vi "transferPrivate.vi"(8 "error in (no error)":errorcluster, 10 "TransferFrom in":refnum<class "xceNode.lvclass">, 11 "TransferTo in":refnum<class "xceDataNode.lvclass">) -> (0 "error out":errorcluster, 2 "TransferFrom out":refnum<class "xceNode.lvclass">, 3 "TransferTo out":refnum<class "xceDataNode.lvclass">)   [LabVIEW 2013, in "xceDataNode.lvclass"]
doc: "Transfers all private data from one xceDataNode to another. Used primarily to replace a node with another in the tree data structure."
uses:
  xceDataNode.lvclass
  xceNode/xceNode.lvclass
  xceDataNode.lvclass/xceDataNode.ctl
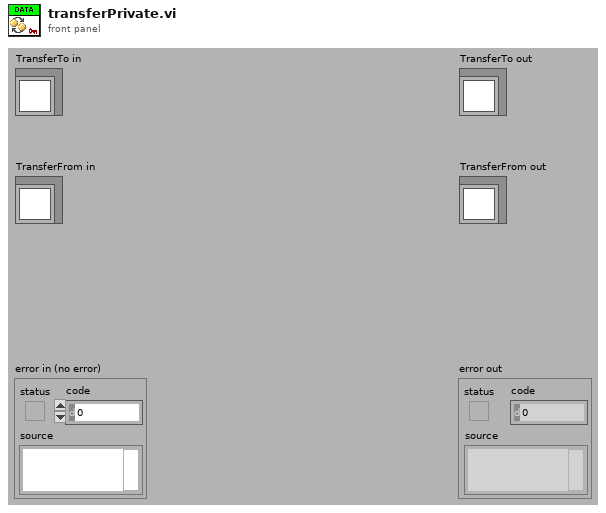
[diagram p1: front panel]
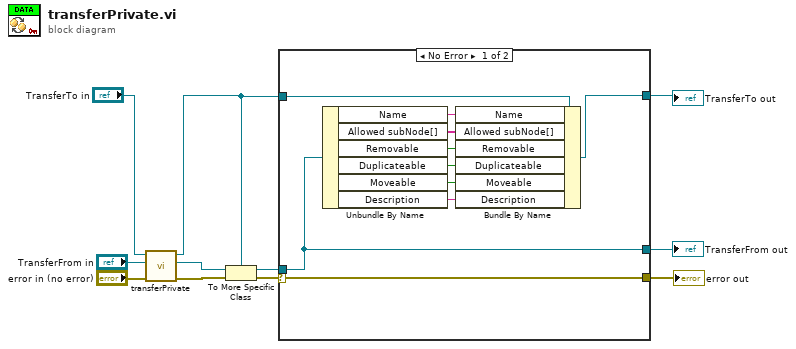
[diagram p0: block diagram]
diagram:
  n1 = call-parent "transferPrivate.vi"("error in (no error)"="error in (no error)", "TransferFrom in"="TransferFrom in", "TransferTo in"="TransferTo in") -> ("error out"=w7:errorcluster, "TransferFrom out"=w8:refnum<class "xceNode.lvclass">, "TransferTo out"=w5:refnum<class "xceDataNode.lvclass">)  [unwired: 6 in]
  n2 = To More Specific Class(target class=w5, reference=w8, error in=w7) -> (specific class reference=w4:refnum<class "xceDataNode.lvclass">, error out=w6:errorcluster)
  n3 = case shown="No Error" w6 {
    selector: w6 -> [w14 w22]
    tunnel: w5 -> [w21 w24]
    tunnel: w4 -> [w13 w23]
    tunnel: [w14 w22] -> w3
    tunnel: [w13 w23] -> w2
    tunnel: [w12 w24] -> w1
    frame No Error {
      n4 = Unbundle By Name(w13) -> ("Name"=w19:string, "Allowed subNode[]"=w18:string[], "Removable"=w20:bool, "Duplicateable"=w17:bool, "Moveable"=w16:bool, "Description"=w15:string)
      n5 = Bundle By Name(cluster=w21, "Name"=w19, "Allowed subNode[]"=w18, "Removable"=w20, "Duplicateable"=w17, "Moveable"=w16, "Description"=w15) -> (w12:refnum<class "xceDataNode.lvclass">)
    }
    frame Error {
    }
  }
  "error out" <- w3
  "TransferTo out" <- w1
  "TransferFrom out" <- w2
